vi "myRIO__convert__Probability_to_TrueFalse.vi"(11 "input_probability_u16":u16) -> (3 "output_TF":bool)   [LabVIEW 2014]
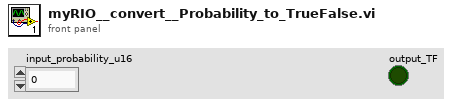
[diagram p1: front panel]
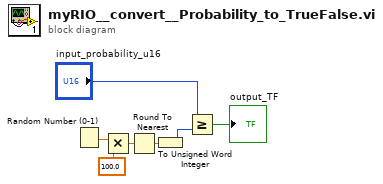
[diagram p0: block diagram]
diagram:
  n1 = Random Number (0-1)() -> (number: 0 to 1=w7:dbl)
  n2 = Multiply(x=w7, y=100.0) -> (x*y=w6:dbl)
  n3 = Round To Nearest(number=w6) -> (nearest integer value=w5:dbl)
  n4 = To Unsigned Word Integer(number=w5) -> (unsigned 16bit integer=w4:u16)
  n5 = Greater Or Equal?(x="input_probability_u16", y=w4) -> (x >= y?=→"output_TF":bool)
